vi "GetPhaseOrderProperties.vi"(8 "error in (no error)":errorcluster, 9 "Channels":T1[](array[typedef]), 10 "Channel Properties":T2[](array[typedef]), 11 "ChannelType":string) -> (0 "error out":errorcluster, 1 "Phase C ChannelName":string, 2 "Phase B ChannelName":string, 3 "Phase A ChannelName":string, 5 "wiring configuraiton":string)   [LabVIEW 2017, in "McsaAnalysisFunctions.lvlib"]
uses:
  <vilib>/addons/InsightCM/Utilities/Analysis/MCSA/McsaAnalysisFunctions.lvlib
  <vilib>/addons/InsightCM/MessageBus/Base/controls/KeyValuePair.ctl
  <vilib>/addons/InsightCM/MessageBus/Base/controls/R2_Channel.ctl
  <vilib>/addons/InsightCM/MessageBus/Base/controls/Metric.ctl
  <vilib>/addons/InsightCM/Utilities/PropertyHelpers/PropertyHelpers.lvlib
  <vilib>/addons/InsightCM/Utilities/MCSA/McsaUtilities.lvlib
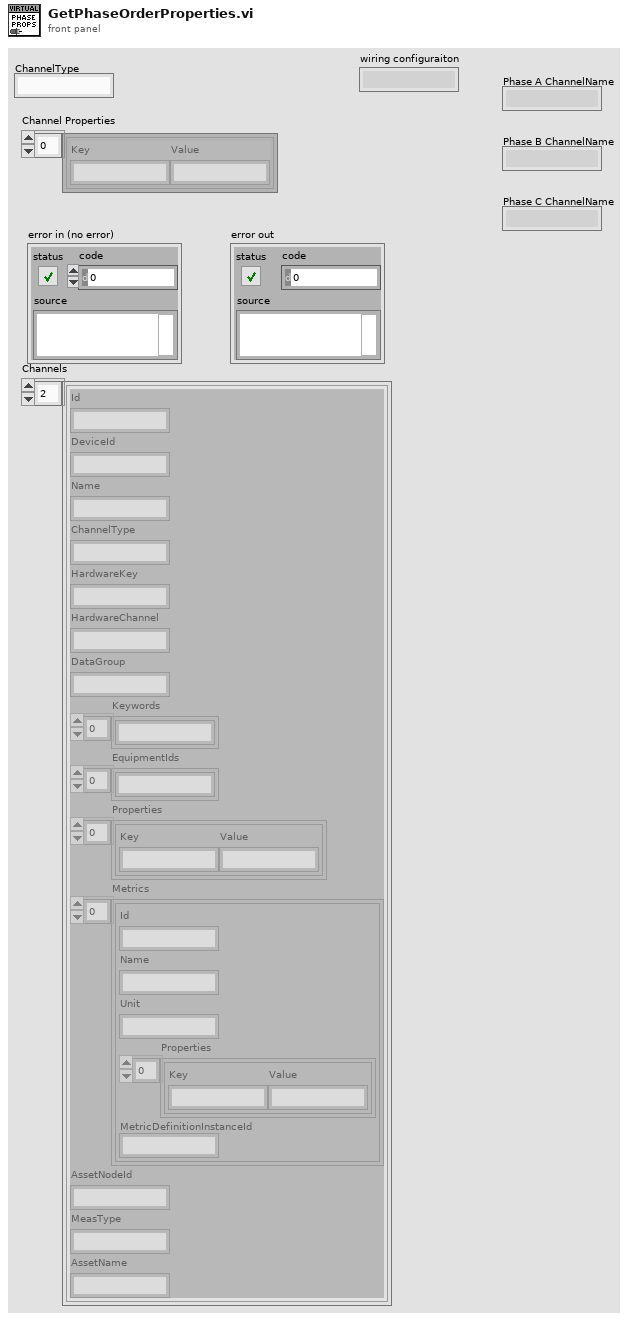
[diagram p1: front panel]
types:
  T1 = typedef "R2_Channel.ctl" = cluster{"Id":string, "DeviceId":string, "Name":string, "ChannelType":string, "HardwareKey":string, "HardwareChannel":string, "DataGroup":string, "Keywords":string[], "EquipmentIds":string[], "Properties":T2[], "Metrics":T3[], "AssetNodeId":string, "MeasType":string, "AssetName":string}
  T2 = typedef "KeyValuePair.ctl" = cluster{"Key":string, "Value":string}
  T3 = typedef "Metric.ctl" = cluster{"Id":string, "Name":string, "Unit":string, "Properties":T2[], "MetricDefinitionInstanceId":string}
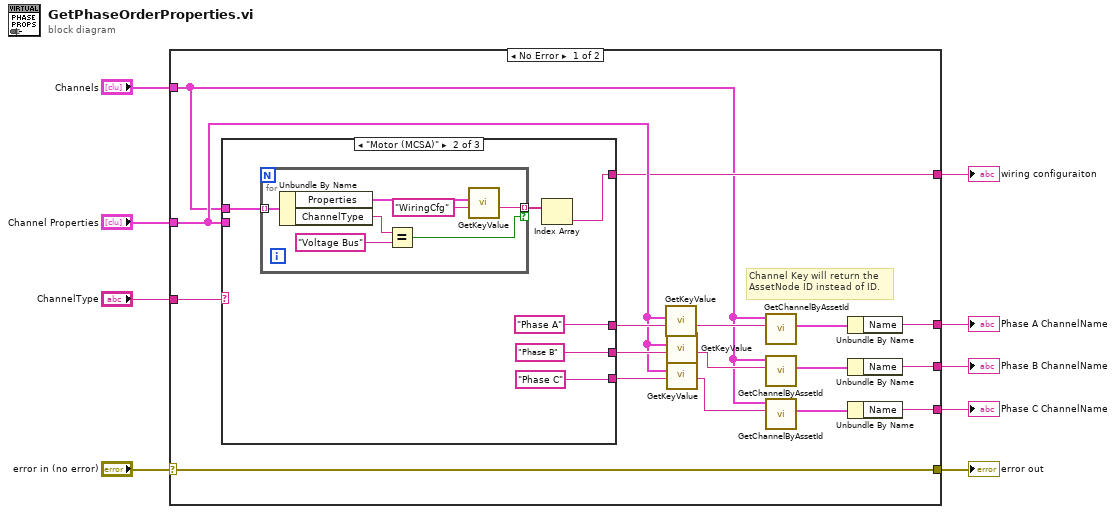
[diagram p0: block diagram]
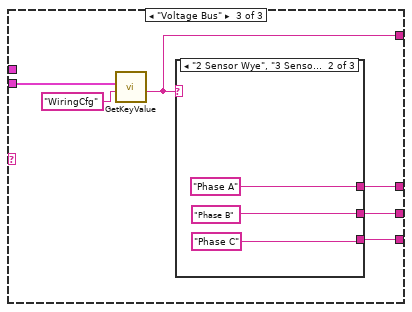
[diagram p3: hidden frame]
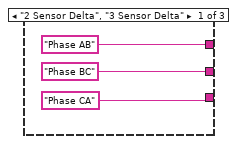
[diagram p4: hidden frame]
diagram:
  n1 = case shown="No Error" "error in (no error)" {
    selector: "error in (no error)" -> [w13 w52]
    tunnel: "ChannelType" -> [w12 _]
    tunnel: "Channels" -> [w10 _]
    tunnel: [w23 _] -> w7
    tunnel: [w22 _] -> w6
    tunnel: [w21 _] -> w5
    tunnel: "Channel Properties" -> [w15 _]
    tunnel: [w13 w52] -> w2
    tunnel: [w11 _] -> w1
    frame No Error {
      # "Channel Key will return the\nAssetNode ID instead of ID."
      n2 = case shown="\"Motor (MCSA)\"" w12 {
        tunnel: w15 -> [_ _ w44]
        tunnel: [_ "Phase C" ("Name") w43] -> w16
        tunnel: [_ "Phase B" ("Name") w42] -> w18
        tunnel: [_ "Phase A" ("Name") w41] -> w20
        tunnel: [_ w28 w40] -> w11
        tunnel: w10 -> [_ w27 _]
        frame Default {
        }
        frame "Motor (MCSA)" {
          n3 = for {
            tunnel: w27 -> [w39] mode=indexing
            tunnel: [w34] -> w29 mode=indexing if=w33
            n4 = Unbundle By Name(w39) -> ("Properties"=w38:T2[], "ChannelType"=w36:string)
            n5 = Equal?(x=w36, y="Voltage Bus") -> (x = y?=w33:bool)
            n6 = call <vilib>:"GetKeyValue.vi"("key"="WiringCfg" ("Name"), "key value pairs"=w38) -> ("value"=w34:string)  [unwired: 7 in, 2 out]
          }
          n7 = Index Array(array=w29) -> (element=w28:string)  [unwired: 1 in]
        }
        frame "Voltage Bus" {
          n8 = call <vilib>:"GetKeyValue.vi"("key"="WiringCfg" ("Name"), "key value pairs"=w44) -> ("value"=w40:string)  [unwired: 7 in, 2 out]
          n9 = case shown="\"2 Sensor Wye\", \"3 Sensor Wye\"" w40 {
            tunnel: ["Phase AB" ("Name") "Phase A" ("Name") _] -> w41
            tunnel: ["Phase BC" ("Name") "Phase B" ("Name") _] -> w42
            tunnel: ["Phase CA" ("Name") "Phase C" ("Name") _] -> w43
            frame "2 Sensor Delta", "3 Sensor Delta" {
            }
            frame "2 Sensor Wye", "3 Sensor Wye" {
            }
            frame Default {
            }
          }
        }
      }
      n10 = call <vilib>:"GetKeyValue.vi"("key"=w20, "key value pairs"=w15) -> ("value"=w19:string)  [unwired: 7 in, 2 out]
      n11 = call <vilib>:"GetKeyValue.vi"("key"=w18, "key value pairs"=w15) -> ("value"=w17:string)  [unwired: 7 in, 2 out]
      n12 = call <vilib>:"GetKeyValue.vi"("key"=w16, "key value pairs"=w15) -> ("value"=w14:string)  [unwired: 7 in, 2 out]
      n13 = call <vilib>:"GetChannelByAssetId.vi"("node id"=w19, "channels in"=w10) -> ("channel"=w26:T1)  [unwired: 7 in, 2 out]
      n14 = call <vilib>:"GetChannelByAssetId.vi"("node id"=w17, "channels in"=w10) -> ("channel"=w25:T1)  [unwired: 7 in, 2 out]
      n15 = call <vilib>:"GetChannelByAssetId.vi"("node id"=w14, "channels in"=w10) -> ("channel"=w24:T1)  [unwired: 7 in, 2 out]
      n16 = Unbundle By Name(w26) -> ("Name"=w22:string)
      n17 = Unbundle By Name(w25) -> ("Name"=w23:string)
      n18 = Unbundle By Name(w24) -> ("Name"=w21:string)
    }
    frame Error {
    }
  }
  "error out" <- w2
  "Phase A ChannelName" <- w6
  "Phase B ChannelName" <- w7
  "Phase C ChannelName" <- w5
  "wiring configuraiton" <- w1
